vi "Flush Control Value.vi"(4 "error in (no error)":errorcluster, 5 "Tab Control Ref In":T1, 6 "ActiveAttribute":string, 7 "Session In":T2) -> (0 "error out":errorcluster, 3 "Session Out":T2)   [LabVIEW 2014, in "Camera Quick Settings Panel.lvlib" / "Camera Quick Settings Panel.lvclass"]
doc: "The Flush Control Value subVI reads the value of the control, and then sets the value of the attribute in the IMAQdx driver."
uses:
  Camera Quick Settings Panel.lvclass
  <vilib>/userdefined/High Color/IMAQdx.ctl
  <vilib>/vision/driver/IMAQdx.llb/IMAQdx Attribute Type.ctl
  <resource>/objmgr/imaqdx.rc
  <vilib>/vision/driver/NI_Vision_Acquisition_Software.lvlib
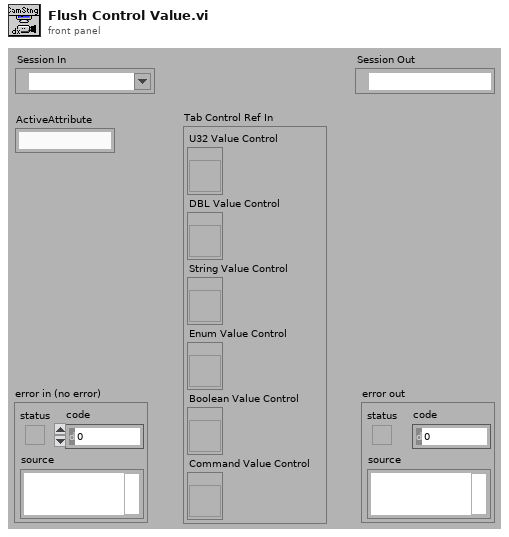
[diagram p1: front panel]
types:
  T1 = cluster{"U32 Value Control":refnum<vi>, "DBL Value Control":refnum<vi>, "String Value Control":refnum<vi>, "Enum Value Control":refnum<vi>, "Boolean Value Control":refnum<vi>, "Command Value Control":refnum<vi>}
  T2 = typedef "IMAQdx.ctl" = refnum<k21>
  T3 = typedef "NI_Vision_Acquisition_Software.lvlib/IMAQdx Attribute Type.ctl" = enum32{"U32", "I64", "DBL", "String", "Enum", "Bool", "Command"}
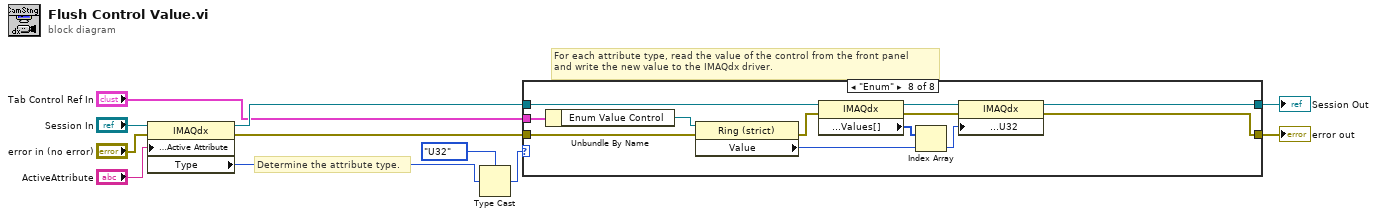
[diagram p0: block diagram]
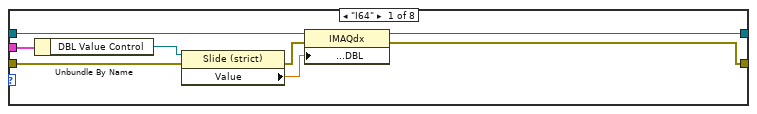
[diagram p2: hidden frame]
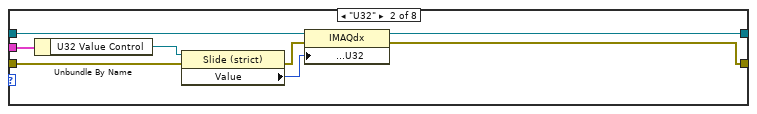
[diagram p3: hidden frame]
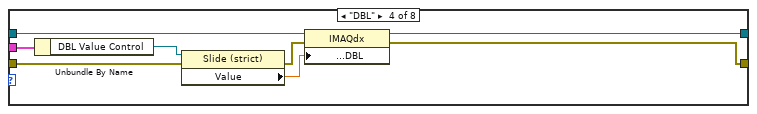
[diagram p5: hidden frame]
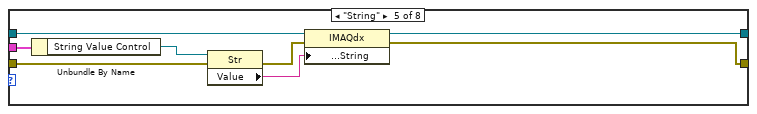
[diagram p6: hidden frame]
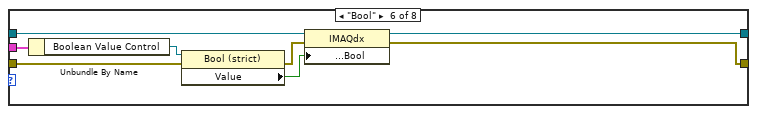
[diagram p7: hidden frame]
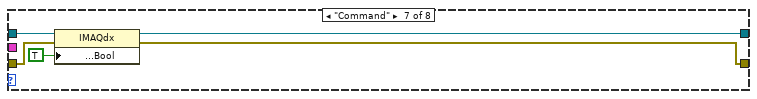
[diagram p8: hidden frame]
diagram:
  # "For each attribute type, read the value of the control from the front panel\nand write the new value to the IMAQdx driver."
  # "Determine the attribute type."
  n1 = property class="IMAQdx"(reference="Session In", error in="error in (no error)", "Camera Attributes:Active Attribute"="ActiveAttribute") -> (reference out=w8:T2, error out=w9:errorcluster, "Type"=w2:u32)
  n2 = Type Cast(type=IMAQdx_Attribute_Type."U32" ("Attribute Type"), x=w2) -> (*(type *) &x=w1:T3)
  n3 = case shown="\"Enum\"" w1 {
    tunnel: w9 -> [w17 w25 w28 w35 w43 w51 w55 w68]
    tunnel: w8 -> [w15 w23 w29 w33 w41 w49 w58 w66]
    tunnel: "Tab Control Ref In" -> [w19 w27 _ w37 w45 w53 _ w70]
    tunnel: [w13 w21 w29 w31 w39 w47 w57 w65] -> w6
    tunnel: [w12 w20 w28 w30 w38 w46 w56 w64] -> w5
    frame "I64" {
      n4 = Unbundle By Name(w19) -> ("DBL Value Control"=w18:refnum<vi>)
      n5 = property class="Slide (strict)"(reference=w18, error in=w17) -> (error out=w16:errorcluster, "Value"=w14:dbl)  [unwired: 1 out]
      n6 = property class="IMAQdx"(reference=w15, error in=w16, "Camera Attributes:Value:DBL"=w14) -> (reference out=w13:T2, error out=w12:errorcluster)
    }
    frame "U32" {
      n7 = Unbundle By Name(w27) -> ("U32 Value Control"=w26:refnum<vi>)
      n8 = property class="Slide (strict)"(reference=w26, error in=w25) -> (error out=w24:errorcluster, "Value"=w22:u32)  [unwired: 1 out]
      n9 = property class="IMAQdx"(reference=w23, error in=w24, "Camera Attributes:Value:U32"=w22) -> (reference out=w21:T2, error out=w20:errorcluster)
    }
    frame Default {
    }
    frame "DBL" {
      n10 = Unbundle By Name(w37) -> ("DBL Value Control"=w36:refnum<vi>)
      n11 = property class="Slide (strict)"(reference=w36, error in=w35) -> (error out=w34:errorcluster, "Value"=w32:dbl)  [unwired: 1 out]
      n12 = property class="IMAQdx"(reference=w33, error in=w34, "Camera Attributes:Value:DBL"=w32) -> (reference out=w31:T2, error out=w30:errorcluster)
    }
    frame "String" {
      n13 = Unbundle By Name(w45) -> ("String Value Control"=w44:refnum<vi>)
      n14 = property class="Str"(reference=w44, error in=w43) -> (error out=w42:errorcluster, "Value"=w40:string)  [unwired: 1 out]
      n15 = property class="IMAQdx"(reference=w41, error in=w42, "Camera Attributes:Value:String"=w40) -> (reference out=w39:T2, error out=w38:errorcluster)
    }
    frame "Bool" {
      n16 = Unbundle By Name(w53) -> ("Boolean Value Control"=w52:refnum<vi>)
      n17 = property class="Bool (strict)"(reference=w52, error in=w51) -> (error out=w50:errorcluster, "Value"=w48:bool)  [unwired: 1 out]
      n18 = property class="IMAQdx"(reference=w49, error in=w50, "Camera Attributes:Value:Bool"=w48) -> (reference out=w47:T2, error out=w46:errorcluster)
    }
    frame "Command" {
      n19 = property class="IMAQdx"(reference=w58, error in=w55, "Camera Attributes:Value:Bool"=TRUE ("ValueBool")) -> (reference out=w57:T2, error out=w56:errorcluster)
    }
    frame "Enum" {
      n20 = Unbundle By Name(w70) -> ("Enum Value Control"=w69:refnum<vi>)
      n21 = property class="Ring (strict)"(reference=w69, error in=w68) -> (error out=w67:errorcluster, "Value"=w59:u32)  [unwired: 1 out]
      n22 = property class="IMAQdx"(reference=w66, error in=w67) -> (reference out=w63:T2, error out=w62:errorcluster, "Camera Attributes:Enum:Values[]"=w61:u32[])
      n23 = Index Array(array=w61, index=w59) -> (element=w60:u32)
      n24 = property class="IMAQdx"(reference=w63, error in=w62, "Camera Attributes:Value:U32"=w60) -> (reference out=w65:T2, error out=w64:errorcluster)
    }
  }
  "Session Out" <- w6
  "error out" <- w5
